vi "TCP_M 서버.vi"() -> ()   [LabVIEW 2018]
uses:
  TypeDefine/Server Status.ctl
panel:
  out "Current Data":dbl
  in  "정지":bool
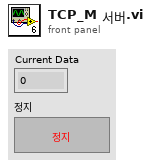
[diagram p1: front panel]
types:
  T1 = typedef "Server Status.ctl" = enum16{"초기화", "Listen and Connect", "Send Data", "Stop"}
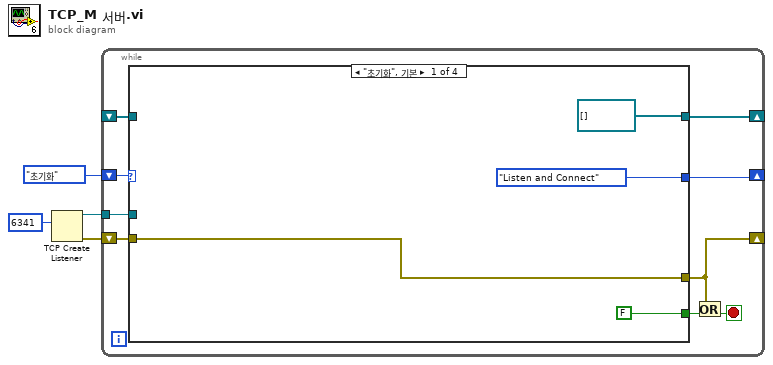
[diagram p0: block diagram]
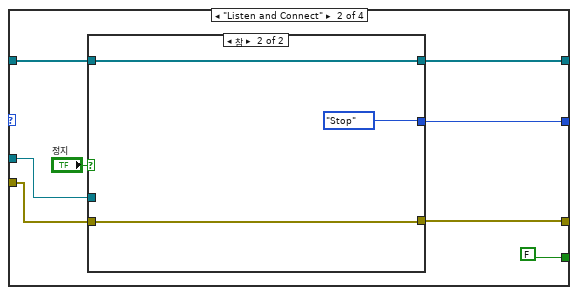
[diagram p2: hidden frame]
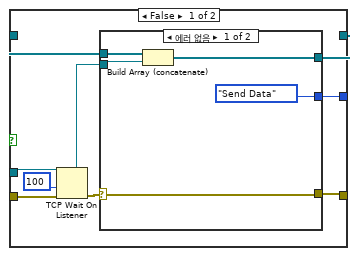
[diagram p3: hidden frame]
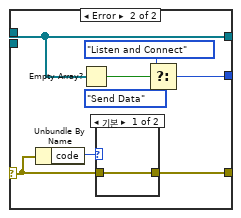
[diagram p4: hidden frame]
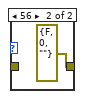
[diagram p5: hidden frame]
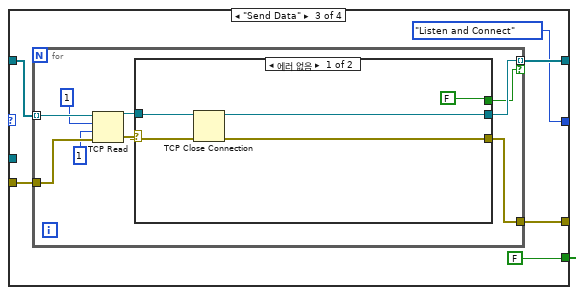
[diagram p6: hidden frame]
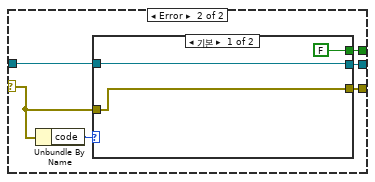
[diagram p7: hidden frame]
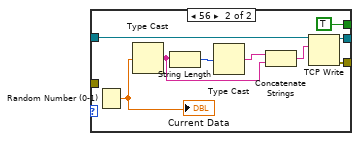
[diagram p8: hidden frame]
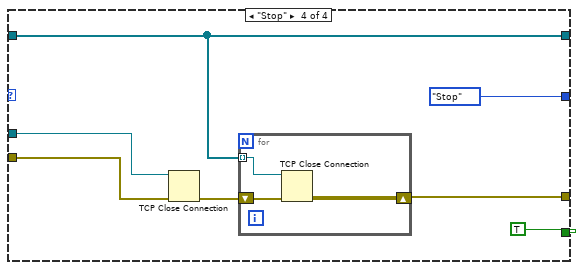
[diagram p9: hidden frame]
diagram:
  n1 = TCP Create Listener(10:u16 6341 ("포트")) -> (0:w3:errorcluster, 3:w2:refnum<k5>)  [unwired: 4 in, 1 out]
  n2 = while {
    shift-right: [w12] -> _
    shift-left: Server_Status."초기화" ("열거형") -> [w13]
    shift-right: [w8] -> _
    shift-left: w3 -> [w10]
    tunnel: w2 -> [w11]
    shift-right: [w5] -> _
    shift-left: _ -> [w6]
    stop <- w7 stop-if-true
    n3 = case shown="\"초기화\", 기본" w13 {
      tunnel: [Server_Status."Listen and Connect" ("열거형") w20 Server_Status."Listen and Connect" ("열거형") Server_Status."Stop" ("열거형")] -> w12
      tunnel: w11 -> [_ w22 _ w97]
      tunnel: [w16 w21 w55 w93] -> w8
      tunnel: w10 -> [w16 w18 w58 w96]
      tunnel: [FALSE FALSE FALSE TRUE] -> w9
      tunnel: w6 -> [_ w24 w57 w95]
      tunnel: [refnum<k5>[] [] w23 w56 w95] -> w5
      frame "초기화", Default {
      }
      frame "Listen and Connect" {
        n4 = case shown="참" "정지" {
          tunnel: [w28 w52] -> w23
          tunnel: w24 -> [w29 w52]
          tunnel: w22 -> [w34 _]
          tunnel: [w30 w51] -> w21
          tunnel: w18 -> [w33 w51]
          tunnel: [w26 Server_Status."Stop" ("열거형")] -> w20
          frame False {
            n5 = TCP Wait On Listener(8:w33, 9:100 ("타임아웃 ms (계속 기다림: -1)"), 11:w34) -> (0:w31:errorcluster, 4:w27:refnum<k5>)  [unwired: 1 in, 3 out]
            n6 = case shown="에러 없음" w31 {
              selector: w31 -> [w39 w46]
              tunnel: [w39 w45] -> w30
              tunnel: w29 -> [w38 w42]
              tunnel: [w37 w42] -> w28
              tunnel: w27 -> [w36 _]
              tunnel: [Server_Status."Send Data" ("열거형") w43] -> w26
              frame No Error {
                n7 = Build Array (concatenate)(w38, w36) -> (w37:refnum<k5>[])
              }
              frame Error {
                n8 = Unbundle By Name(w46) -> ("code"=w47:i32)
                n9 = Empty Array?(array=w42) -> (empty?=w44:bool)
                n10 = case shown="기본" w47 {
                  tunnel: w46 -> [w48 _]
                  tunnel: [w48 errorcluster {"status"=FALSE, "code"=0, "source"=""} ("에러 상수")] -> w45
                  frame Default {
                  }
                  frame 56 {
                  }
                }
                n11 = Select(t=Server_Status."Listen and Connect" ("열거형"), s=w44, f=Server_Status."Send Data" ("열거형")) -> (s? t:f=w43:T1)
              }
            }
          }
          frame True {
          }
        }
      }
      frame "Send Data" {
        n12 = for {
          tunnel: w58 -> [w67]
          tunnel: w57 -> [w66] mode=indexing
          tunnel: [w61] -> w56 mode=indexing if=w59
          tunnel: [w60] -> w55
          n13 = TCP Read(connection ID=w66, bytes to read=1 ("읽을 바이트"), error in (no error)=w67, 9:1 ("타임아웃 ms (25000)")) -> (connection ID out=w62:refnum<k5>, error out=w63:errorcluster)  [unwired: 1 in, 1 out]
          n14 = case shown="에러 없음" w63 {
            selector: w63 -> [w71 w78]
            tunnel: w62 -> [w72 w76]
            tunnel: [w69 w75] -> w61
            tunnel: [w70 w74] -> w60
            tunnel: [FALSE w73] -> w59
            frame No Error {
              n15 = TCP Close Connection(connection ID=w72, error in (no error)=w71) -> (connection ID out=w69:refnum<k5>, error out=w70:errorcluster)  [unwired: 1 in]
            }
            frame Error {
              n16 = Unbundle By Name(w78) -> ("code"=w77:i32)
              n17 = case shown="기본" w77 {
                tunnel: w78 -> [w81 _]
                tunnel: w76 -> [w80 w90]
                tunnel: [w80 w84] -> w75
                tunnel: [w81 w83] -> w74
                tunnel: [FALSE TRUE] -> w73
                frame Default {
                }
                frame 56 {
                  n18 = Random Number (0-1)() -> (number: 0 to 1=w89:dbl)
                  "Current Data" <- w89
                  n19 = Type Cast(x=w89) -> (*(type *) &x=w86:string)  [unwired: 1 in]
                  n20 = String Length(string=w86) -> (length=w88:i32)
                  n21 = Type Cast(x=w88) -> (*(type *) &x=w87:string)  [unwired: 1 in]
                  n22 = Concatenate Strings(w87, w86) -> (w85:string)
                  n23 = TCP Write(connection ID=w90, data in=w85) -> (connection ID out=w84:refnum<k5>, error out=w83:errorcluster)  [unwired: 2 in, 1 out]
                }
              }
            }
          }
        }
      }
      frame "Stop" {
        n24 = TCP Close Connection(connection ID=w97, error in (no error)=w96) -> (error out=w94:errorcluster)  [unwired: 1 in, 1 out]
        n25 = for {
          tunnel: w95 -> [w98] mode=indexing
          shift-right: [w99] -> w93
          shift-left: w94 -> [w100]
          n26 = TCP Close Connection(connection ID=w98, error in (no error)=w100) -> (error out=w99:errorcluster)  [unwired: 1 in, 1 out]
        }
      }
    }
    n27 = Or(x=w8, y=w9) -> (x .or. y?=w7:bool)
  }
